vi "Igor_StringArraytoIgorWave.vi"(8 "error in (no error)":errorcluster, 10 "Wave":string[](array[string]), 11 "Name":string) -> (0 "error out":errorcluster, 3 "Igor Wave":string)   [LabVIEW 2019]
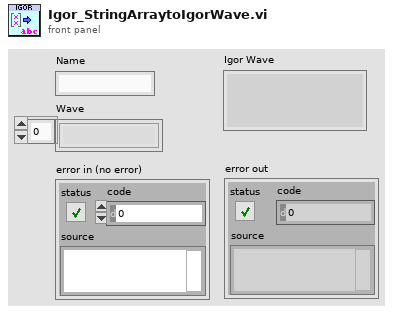
[diagram p1: front panel]
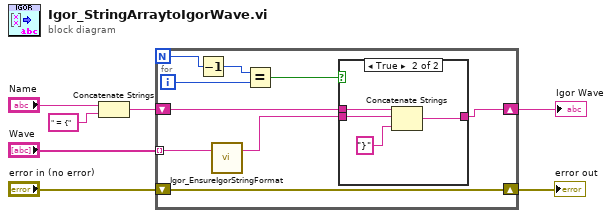
[diagram p0: block diagram]
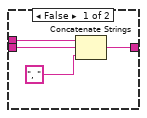
[diagram p2: hidden frame]
diagram:
  n1 = Concatenate Strings("Name", " = {" ("string")) -> (w5:string)
  n2 = for {
    N -> [w14]
    tunnel: "Wave" -> [w10] mode=indexing
    shift-right: [w15] -> w4
    shift-left: w5 -> [w16]
    shift-right: [w8] -> w2
    shift-left: "error in (no error)" -> [w8]
    i -> [w12]
    n3 = Decrement(x=w14) -> (x-1=w13:i32)
    n4 = call "Igor_EnsureIgorStringFormat.vi"("Value"=w10) -> ("Value"=w9:string)  [unwired: 2 in]
    n5 = Equal?(x=w13, y=w12) -> (x = y?=w11:bool)
    n6 = case shown="True" w11 {
      tunnel: w16 -> [w20 w24]
      tunnel: w9 -> [w19 w23]
      tunnel: [w17 w21] -> w15
      frame False {
        n7 = Concatenate Strings(w20, w19, ", " ("string")) -> (w17:string)
      }
      frame True {
        n8 = Concatenate Strings(w24, w23, "}") -> (w21:string)
      }
    }
  }
  "error out" <- w2
  "Igor Wave" <- w4
